vi "Resolve Variant.vi"(8 "error in (no error)":errorcluster, 10 "Value":variant, 11 "Promise in":refnum<class "Promise.lvclass">) -> (0 "error out":errorcluster, 3 "Promise out":refnum<class "Promise.lvclass">)   [LabVIEW 2020, in "Promises.lvlib" / "Promise.lvclass"]
uses:
  Promise.lvclass
  Promise.lvclass/Promise.ctl
  Variant/Variant.lvclass
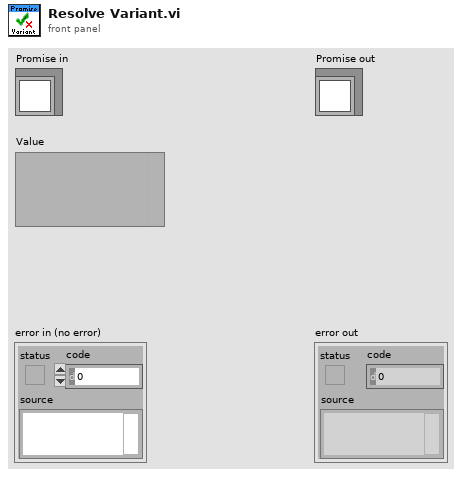
[diagram p1: front panel]
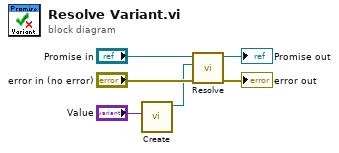
[diagram p0: block diagram]
diagram:
  n1 = call "Create.vi"("Value"="Value") -> ("Variant out"=w1:refnum<class "Variant.lvclass">)  [unwired: 10 in]
  n2 = call "Resolve.vi"("error in (no error)"="error in (no error)", "Result (None)"=w1, "Promise in"="Promise in") -> ("error out"=→"error out":errorcluster, "Promise out"=→"Promise out":refnum<class "Promise.lvclass">)  [unwired: 7 in]
